vi "Create Map of VI and Lib Ref.vi"(8 "error in":errorcluster caption="error out", 9 "RT Target":bool=TRUE, 11 "VI and Library References":T1[](array[typedef])) -> (0 "error out":errorcluster, 2 "Library Map":map{string, refnum<vi>}(c390), 3 "VI Map":map{string, refnum<vi>}(c390))   [LabVIEW 2021, in "LV Scripting Utilities.lvlib"]
uses:
  LV Scripting Utilities.lvlib
  <vilib>/Utility/EditLVProj/Library And VI References.ctl
  <vilib>/Utility/EditLVProj/Edit LVProj.lvlib
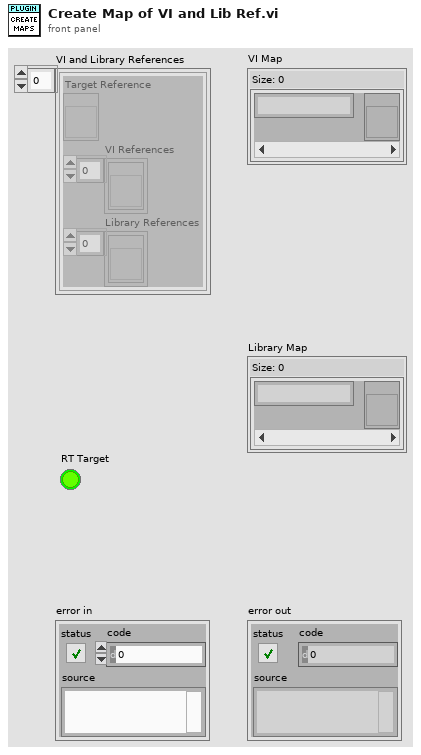
[diagram p1: front panel]
types:
  T1 = typedef "Edit LVProj.lvlib/Library And VI References.ctl" = cluster{"Target Reference":refnum<vi>, "VI References":refnum<vi>[], "Library References":refnum<vi>[]}
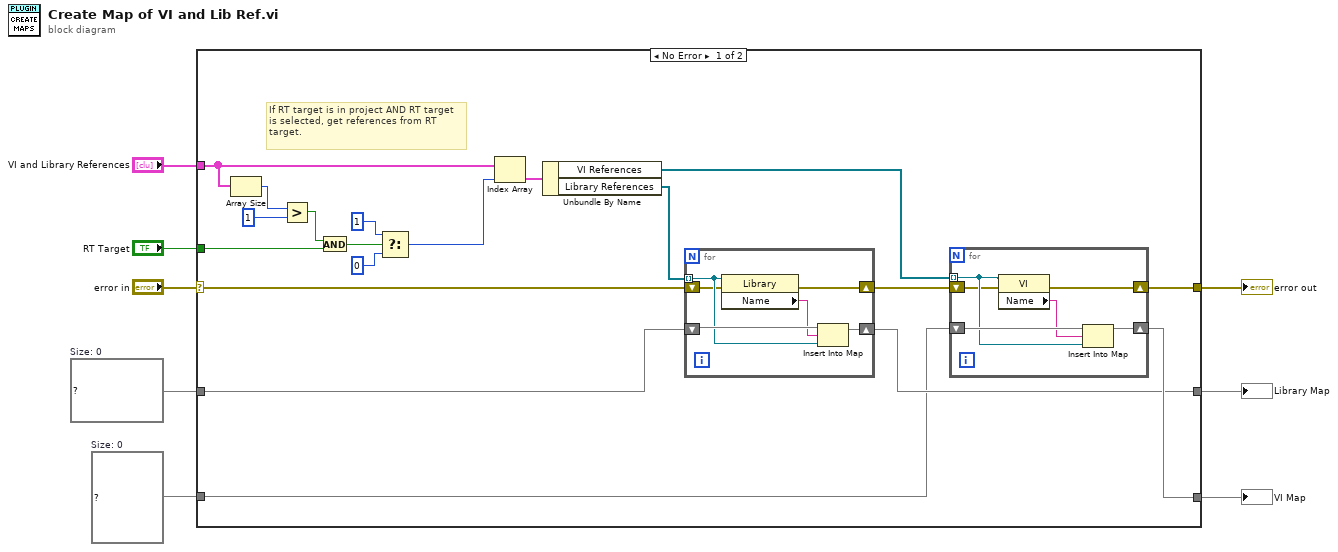
[diagram p0: block diagram]
diagram:
  w1 = map{string, refnum<vi>} {}  # Size: 0
  w2 = map{string, refnum<vi>} {}  # Size: 0
  n1 = case shown="No Error" "error in" {
    selector: "error in" -> [w11 w42]
    tunnel: "VI and Library References" -> [w24 _]
    tunnel: [w14 w42] -> w6
    tunnel: "RT Target" -> [w20 _]
    tunnel: [w13 w40] -> w4
    tunnel: [w12 w41] -> w3
    tunnel: w2 -> [w10 w41]
    tunnel: w1 -> [w9 w40]
    frame No Error {
      # "If RT target is in project AND RT target is selected, get references from RT target."
      n2 = Array Size(array=w24) -> (size(s)=w23:i32)
      n3 = Greater?(x=w23, y=1) -> (0:w21:bool)
      n4 = And(x=w21, y=w20) -> (x .and. y?=w19:bool)
      n5 = Select(t=1 ("index"), s=w19, f=0 ("index")) -> (s? t:f=w18:i32)
      n6 = Index Array(array=w24, index=w18) -> (element=w27:T1)
      n7 = Unbundle By Name(w27) -> ("VI References"=w25:refnum<vi>[], "Library References"=w26:refnum<vi>[])
      n8 = for {
        shift-right: [w38] -> w12
        shift-left: w10 -> [w39]
        tunnel: w26 -> [w36] mode=indexing
        shift-right: [w35] -> w15
        shift-left: w11 -> [w34]
        n9 = property class="Library"(reference=w36, error in=w34) -> (error out=w35:errorcluster, "Name"=w37:string)  [unwired: 1 out]
        n10 = Insert Into Map(map in=w39, key=w37, value=w36) -> (map out=w38:map{string, refnum<vi>})  [unwired: 2 out]
      }
      n11 = for {
        shift-right: [w32] -> w13
        shift-left: w9 -> [w33]
        tunnel: w25 -> [w31] mode=indexing
        shift-right: [w29] -> w14
        shift-left: w15 -> [w28]
        n12 = property class="VI"(reference=w31, error in=w28) -> (error out=w29:errorcluster, "Name"=w30:string)  [unwired: 1 out]
        n13 = Insert Into Map(map in=w33, key=w30, value=w31) -> (map out=w32:map{string, refnum<vi>})  [unwired: 2 out]
      }
    }
    frame Error {
    }
  }
  "error out" <- w6
  "VI Map" <- w4
  "Library Map" <- w3
